vi "Mono Full Example.vi"(4 "Stop Grating Check":bool, 5 "Stop Position Check":bool, 6 "Stop Init Check":bool, 7 "Stop Move Mirror Check":bool, 8 "error in (no error)":errorcluster, 9 "Stop Slit Check":bool) -> (0 "error out":errorcluster, 3 "config data":T1)   [LabVIEW 2020, in "Examples.lvlib"]
doc: "Overview of the full capabilites of the monochromator."
uses:
  Examples.lvlib
  Classes/Mono/Monochromator.lvclass
  5e8b4889-da11-473e-b5b8-b20730483063.vi
  5fed84ad-8a5e-403e-aaf1-ae4b1277c373.vi
  132430fe-3055-42ba-b41e-c0cbb81a5c5b.vi
  d08bdf09-0d91-431c-977a-345d7eb55896.vi
  5b0376ad-d4d0-4b95-ac3e-4f2238ad5595.vi
  6c06501c-fbb7-40a9-83fb-7bb36eab80cd.vi
  6bd0f17a-df95-4643-b232-1a9d4f6286d3.vi
  f58601d0-aaf6-4926-8fdd-c6ddc7369c5d.vi
  43362571-0f95-4bd5-9137-2acaa5e1e114.vi
  caaad9aa-0ae1-44e5-9847-f9e0e622223b.vi
  Classes/Mono/filterWheel.ctl
  Classes/Mono/grating.ctl
  Classes/Mono/mirror.ctl
  Classes/Mono/port.ctl
  Classes/Mono/configuration.ctl
panel:
  out "new position":dbl
  out "position":dbl
  out "shutterPosition":i32
  out "shutterIndex":i32
  out "wavelength":dbl
  out "new wavelength":dbl format="%.2f"
  out "new Mirror Position":i32
  out "Mirror Position":i32
  out "new is initialized?":bool
  out "mono is initialized?":bool
  out "new Grating Position":i32
  out "Grating Position":i32
  out "filterWheelPosition":i32
  # "Connector Pane"
  # "Locals"
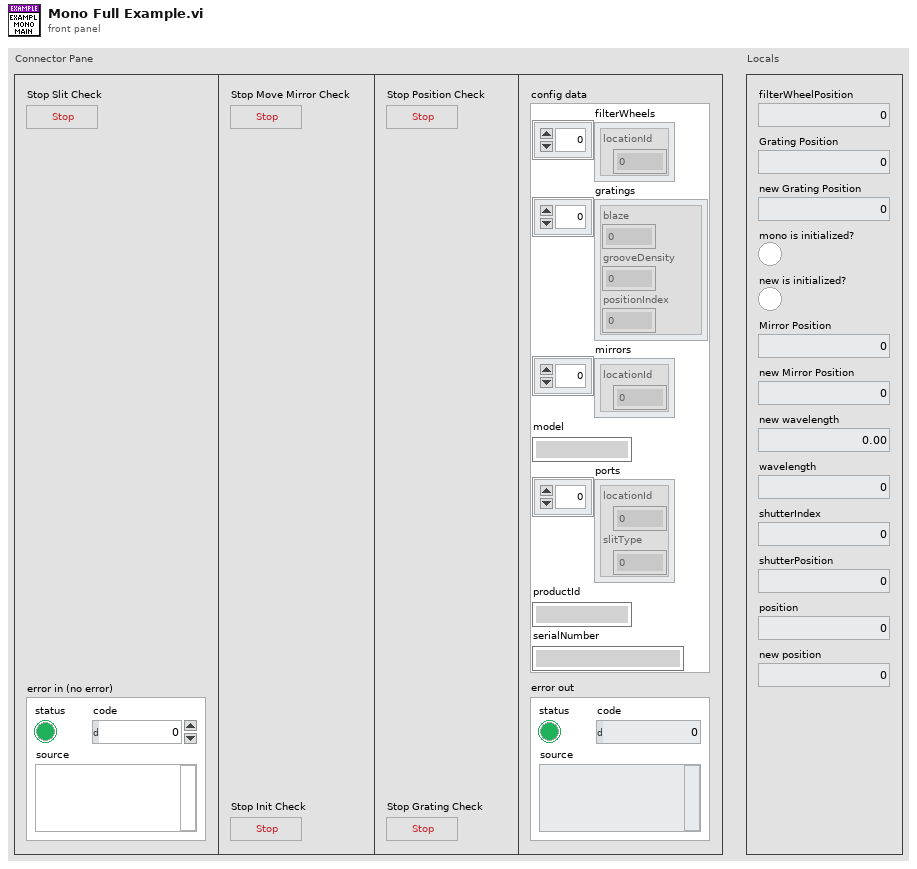
[diagram p1: front panel]
types:
  T1 = typedef "horiba.lvlib/Monochromator.lvclass/configuration.ctl" = cluster{"filterWheels":T2[], "gratings":T3[], "mirrors":T4[], "model":string, "ports":T5[], "productId":string, "serialNumber":string}
  T2 = typedef "horiba.lvlib/Monochromator.lvclass/filterWheel.ctl" = cluster{"locationId":i32}
  T3 = typedef "horiba.lvlib/Monochromator.lvclass/grating.ctl" = cluster{"blaze":i32, "grooveDensity":i32, "positionIndex":i32}
  T4 = typedef "horiba.lvlib/Monochromator.lvclass/mirror.ctl" = cluster{"locationId":i32}
  T5 = typedef "horiba.lvlib/Monochromator.lvclass/port.ctl" = cluster{"locationId":i32, "slitType":i32}
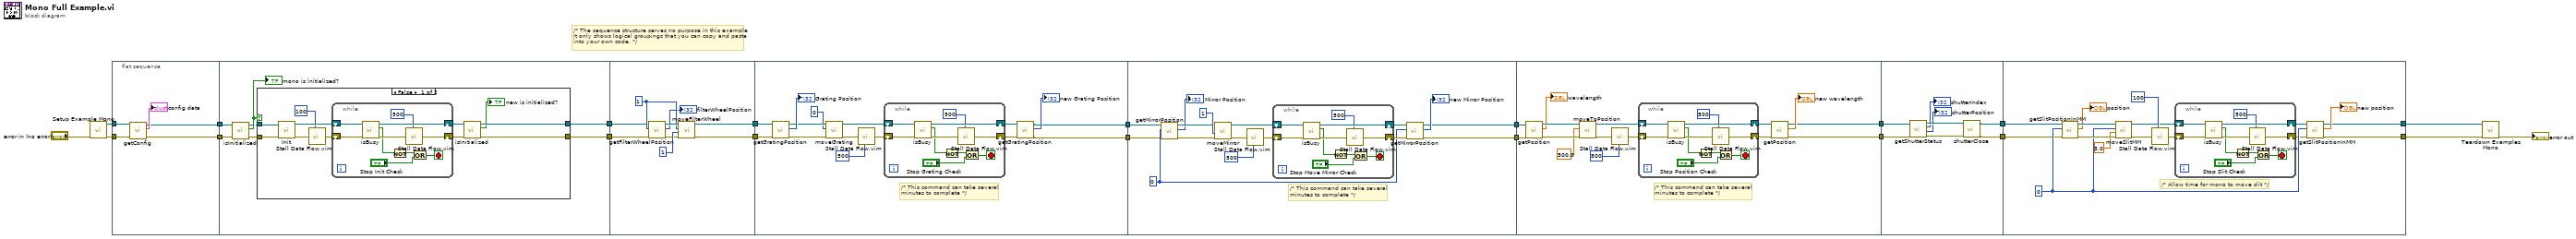
[diagram p0: block diagram]
diagram:
  # "/* The sequence structure serves no purpose in this example\nIt only shows logical groupings that you can copy and paste \ninto your own code. */"
  n1 = call "Setup Example Mono.vi"("error in (no error)"="error in (no error)") -> ("error out"=w19:errorcluster, "Mono Out"=w20:refnum<class "Monochromator.lvclass">)  [unwired: 7 in, 2 out]
  n2 = flat-sequence {
    tunnel: w20 -> [w25]
    tunnel: w19 -> [w24]
    tunnel: [w22] -> w14
    tunnel: [w21] -> w12
    tunnel: w14 -> [w29]
    tunnel: [w26] -> w13
    tunnel: w12 -> [w28]
    tunnel: [w27] -> w11
    tunnel: w13 -> [w59]
    tunnel: w11 -> [w58]
    tunnel: [w57] -> w16
    tunnel: [w56] -> w15
    tunnel: w16 -> [w68]
    tunnel: w15 -> [w67]
    tunnel: [w66] -> w10
    tunnel: [w65] -> w9
    tunnel: w10 -> [w93]
    tunnel: w9 -> [w92]
    tunnel: [w91] -> w8
    tunnel: [w90] -> w7
    tunnel: w8 -> [w119]
    tunnel: w7 -> [w118]
    tunnel: [w117] -> w6
    tunnel: [w116] -> w5
    tunnel: w6 -> [w144]
    tunnel: w5 -> [w143]
    tunnel: [w142] -> w4
    tunnel: [w141] -> w3
    tunnel: w4 -> [w152]
    tunnel: w3 -> [w151]
    tunnel: [w150] -> w2
    tunnel: [w149] -> w1
    frame #0 {
      n3 = call "getConfig.vi"("error in (no error)"=w24, "Monochromator in"=w25) -> ("error out"=w22:errorcluster, "config data"=→"config data":T1, "Monochromator out"=w21:refnum<class "Monochromator.lvclass">)  [unwired: 6 in, 1 out]
    }
    frame #1 {
      n4 = call "isInitialized.vi"("error in (no error)"=w29, "Monochromator in"=w28) -> ("error out"=w31:errorcluster, "mono is initialized?"=w32:bool, "Monochromator out"=w30:refnum<class "Monochromator.lvclass">)  [unwired: 7 in]
      "mono is initialized?" <- w32
      n5 = case shown="False" w32 {
        tunnel: [w41 w55] -> w26
        tunnel: [w40 w54] -> w27
        tunnel: w31 -> [w34 w55]
        tunnel: w30 -> [w33 w54]
        frame False {
          n6 = call "Init.vi"("error in (no error)"=w34, "Monochromator in"=w33) -> ("error out"=w43:errorcluster, "Monochromator out"=w42:refnum<class "Monochromator.lvclass">)  [unwired: 6 in, 2 out]
          n7 = call "Stall Data Flow.vim"("value in"=w43, "milliseconds to wait"=u32 100) -> ("value out"=w38:errorcluster)  [unwired: 1 out]
          n8 = while {
            shift-right: [w49] -> w36
            shift-left: w38 -> [w51]
            shift-right: [w52] -> w37
            shift-left: w42 -> [w50]
            stop <- w46 stop-if-true
            n9 = call "isBusy.vi"("error in (no error)"=w51, "Monochromator in"=w50) -> ("error out"=w53:errorcluster, "mono is busy?"=w47:bool, "Monochromator out"=w52:refnum<class "Monochromator.lvclass">)  [unwired: 7 in]
            n10 = Not(x=w47) -> (.not. x?=w44:bool)
            n11 = call "Stall Data Flow.vim"("value in"=w53, "milliseconds to wait"=u32 500) -> ("value out"=w49:errorcluster)  [unwired: 1 out]
            n12 = Or(x=w44, y="Stop Init Check") -> (x .or. y?=w46:bool)
          }
          n13 = call "isInitialized.vi"("error in (no error)"=w36, "Monochromator in"=w37) -> ("error out"=w41:errorcluster, "mono is initialized?"=→"new is initialized?":bool, "Monochromator out"=w40:refnum<class "Monochromator.lvclass">)  [unwired: 7 in]
        }
        frame True {
        }
      }
    }
    frame #2 {
      w63 = 1 ("locationId")
      n14 = call "getFilterWheelPosition.vi"("error in (no error)"=w59, "locationId"=w63, "Monochromator in"=w58) -> ("error out"=w60:errorcluster, "position"=→"filterWheelPosition":i32, "Monochromator out"=w64:refnum<class "Monochromator.lvclass">)  [unwired: 6 in]
      n15 = call "moveFilterWheel.vi"("error in (no error)"=w60, "position"=1, "locationId"=w63, "Monochromator in"=w64) -> ("error out"=w56:errorcluster, "Monochromator out"=w57:refnum<class "Monochromator.lvclass">)  [unwired: 4 in, 2 out]
    }
    frame #3 {
      # "/* This command can take several \nminutes to complete */"
      n16 = call "getGratingPosition.vi"("error in (no error)"=w67, "Monochromator in"=w68) -> ("error out"=w77:errorcluster, "Position"=→"Grating Position":i32, "Monochromator out"=w78:refnum<class "Monochromator.lvclass">)  [unwired: 7 in]
      n17 = call "moveGrating.vi"("error in (no error)"=w77, "position"=0, "Monochromator in"=w78) -> ("error out"=w76:errorcluster, "Monochromator out"=w74:refnum<class "Monochromator.lvclass">)  [unwired: 5 in, 2 out]
      n18 = call "Stall Data Flow.vim"("value in"=w76, "milliseconds to wait"=u32 500) -> ("value out"=w75:errorcluster)  [unwired: 1 out]
      n19 = while {
        shift-right: [w85] -> w71
        shift-left: w75 -> [w87]
        shift-right: [w88] -> w72
        shift-left: w74 -> [w86]
        stop <- w82 stop-if-true
        n20 = call "isBusy.vi"("error in (no error)"=w87, "Monochromator in"=w86) -> ("error out"=w89:errorcluster, "mono is busy?"=w83:bool, "Monochromator out"=w88:refnum<class "Monochromator.lvclass">)  [unwired: 7 in]
        n21 = Not(x=w83) -> (.not. x?=w80:bool)
        n22 = call "Stall Data Flow.vim"("value in"=w89, "milliseconds to wait"=u32 500) -> ("value out"=w85:errorcluster)  [unwired: 1 out]
        n23 = Or(x=w80, y="Stop Grating Check") -> (x .or. y?=w82:bool)
      }
      n24 = call "getGratingPosition.vi"("error in (no error)"=w71, "Monochromator in"=w72) -> ("error out"=w65:errorcluster, "Position"=→"new Grating Position":i32, "Monochromator out"=w66:refnum<class "Monochromator.lvclass">)  [unwired: 7 in]
    }
    frame #4 {
      w94 = 0 ("locationId")
      # "/* This command can take several \nminutes to complete */"
      n25 = call "getMirrorPosition.vi"("error in (no error)"=w92, "locationId"=w94, "Monochromator in"=w93) -> ("error out"=w97:errorcluster, "position"=→"Mirror Position":i32, "Monochromator out"=w96:refnum<class "Monochromator.lvclass">)  [unwired: 6 in]
      n26 = call "moveMirror.vi"("error in (no error)"=w97, "position"=1, "Monochromator in"=w96) -> ("error out"=w104:errorcluster, "Monochromator out"=w101:refnum<class "Monochromator.lvclass">)  [unwired: 5 in, 2 out]
      n27 = call "Stall Data Flow.vim"("value in"=w104, "milliseconds to wait"=u32 500) -> ("value out"=w103:errorcluster)  [unwired: 1 out]
      n28 = while {
        shift-right: [w111] -> w98
        shift-left: w103 -> [w113]
        shift-right: [w114] -> w99
        shift-left: w101 -> [w112]
        stop <- w108 stop-if-true
        n29 = call "isBusy.vi"("error in (no error)"=w113, "Monochromator in"=w112) -> ("error out"=w115:errorcluster, "mono is busy?"=w109:bool, "Monochromator out"=w114:refnum<class "Monochromator.lvclass">)  [unwired: 7 in]
        n30 = Not(x=w109) -> (.not. x?=w106:bool)
        n31 = call "Stall Data Flow.vim"("value in"=w115, "milliseconds to wait"=u32 500) -> ("value out"=w111:errorcluster)  [unwired: 1 out]
        n32 = Or(x=w106, y="Stop Move Mirror Check") -> (x .or. y?=w108:bool)
      }
      n33 = call "getMirrorPosition.vi"("error in (no error)"=w98, "locationId"=w94, "Monochromator in"=w99) -> ("error out"=w90:errorcluster, "position"=→"new Mirror Position":i32, "Monochromator out"=w91:refnum<class "Monochromator.lvclass">)  [unwired: 6 in]
    }
    frame #5 {
      # "/* This command can take several \nminutes to complete */"
      n34 = call "getPosition.vi"("error in (no error)"=w118, "Monochromator in"=w119) -> ("error out"=w123:errorcluster, "wavelength"=→"wavelength":dbl, "Monochromator out"=w122:refnum<class "Monochromator.lvclass">)  [unwired: 7 in]
      n35 = call "moveToPosition.vi"("error in (no error)"=w123, "wavelength"=500.0, "Monochromator in"=w122) -> ("error out"=w130:errorcluster, "Monochromator out"=w127:refnum<class "Monochromator.lvclass">)  [unwired: 5 in, 2 out]
      n36 = call "Stall Data Flow.vim"("value in"=w130, "milliseconds to wait"=u32 500) -> ("value out"=w129:errorcluster)  [unwired: 1 out]
      n37 = while {
        shift-right: [w136] -> w124
        shift-left: w129 -> [w138]
        shift-right: [w139] -> w125
        shift-left: w127 -> [w137]
        stop <- w133 stop-if-true
        n38 = call "isBusy.vi"("error in (no error)"=w138, "Monochromator in"=w137) -> ("error out"=w140:errorcluster, "mono is busy?"=w134:bool, "Monochromator out"=w139:refnum<class "Monochromator.lvclass">)  [unwired: 7 in]
        n39 = Not(x=w134) -> (.not. x?=w131:bool)
        n40 = call "Stall Data Flow.vim"("value in"=w140, "milliseconds to wait"=u32 500) -> ("value out"=w136:errorcluster)  [unwired: 1 out]
        n41 = Or(x=w131, y="Stop Position Check") -> (x .or. y?=w133:bool)
      }
      n42 = call "getPosition.vi"("error in (no error)"=w124, "Monochromator in"=w125) -> ("error out"=w116:errorcluster, "wavelength"=→"new wavelength":dbl, "Monochromator out"=w117:refnum<class "Monochromator.lvclass">)  [unwired: 7 in]
    }
    frame #6 {
      n43 = call "getShutterStatus.vi"("error in (no error)"=w143, "Monochromator in"=w144) -> ("error out"=w148:errorcluster, "shutterPosition"=→"shutterPosition":i32, "shutterIndex"=→"shutterIndex":i32, "Monochromator out"=w147:refnum<class "Monochromator.lvclass">)  [unwired: 6 in]
      n44 = call "shutterClose.vi"("error in (no error)"=w148, "Monochromator in"=w147) -> ("error out"=w141:errorcluster, "Monochromator out"=w142:refnum<class "Monochromator.lvclass">)  [unwired: 6 in, 2 out]
    }
    frame #7 {
      w159 = 0 ("locationId")
      # "/* Allow time for mono to move slit */"
      n45 = call "getSlitPositionInMM.vi"("error in (no error)"=w151, "locationId"=w159, "Monochromator in"=w152) -> ("error out"=w164:errorcluster, "position"=→"position":dbl, "Monochromator out"=w163:refnum<class "Monochromator.lvclass">)  [unwired: 6 in]
      n46 = call "moveSlitMM.vi"("error in (no error)"=w164, "position"=3.0, "locationId"=w159, "Monochromator in"=w163) -> ("error out"=w162:errorcluster, "Monochromator out"=w155:refnum<class "Monochromator.lvclass">)  [unwired: 4 in, 2 out]
      n47 = call "Stall Data Flow.vim"("value in"=w162, "milliseconds to wait"=u32 100) -> ("value out"=w156:errorcluster)  [unwired: 1 out]
      n48 = while {
        shift-right: [w170] -> w153
        shift-left: w156 -> [w172]
        shift-right: [w173] -> w154
        shift-left: w155 -> [w171]
        stop <- w167 stop-if-true
        n49 = call "isBusy.vi"("error in (no error)"=w172, "Monochromator in"=w171) -> ("error out"=w174:errorcluster, "mono is busy?"=w168:bool, "Monochromator out"=w173:refnum<class "Monochromator.lvclass">)  [unwired: 7 in]
        n50 = Not(x=w168) -> (.not. x?=w165:bool)
        n51 = call "Stall Data Flow.vim"("value in"=w174, "milliseconds to wait"=u32 500) -> ("value out"=w170:errorcluster)  [unwired: 1 out]
        n52 = Or(x=w165, y="Stop Slit Check") -> (x .or. y?=w167:bool)
      }
      n53 = call "getSlitPositionInMM.vi"("error in (no error)"=w153, "locationId"=w159, "Monochromator in"=w154) -> ("error out"=w150:errorcluster, "position"=→"new position":dbl, "Monochromator out"=w149:refnum<class "Monochromator.lvclass">)  [unwired: 6 in]
    }
  }
  n54 = call "Teardown Examples Mono.vi"("error in (no error)"=w2, "Monochromator in"=w1) -> ("error out"=→"error out":errorcluster)  [unwired: 9 in]
